vi "oa_Check Data for Waveform Reference (N Channels).vi"(0 "resampled signal":cluster{"r0":dbl, "dr":dbl, "Y":dbl[]}[](array[cluster]) {"r0" format="%.2p"; "dr" format="%.2p"; "Y" format="%.2f"}, 1 "reset? (True)":bool=TRUE, 5 "select reference data":T2(ring), 7 "speed profile":T1 {"speed [RPM]" format="%.2f"; "time [s]" format="%.2f"}, 9 "interpolated pulse positions":dbl[](array[numeric]) format="%.2f", 11 "error in (no error)":errorcluster, 12 "even angle references in":cluster{"r0":dbl, "dr":dbl, "Y":dbl[]}[](array[cluster]) {"r0" format="%.2p"; "dr" format="%.2p"; "Y" format="%.2f"}) -> (2 "empty signal?":bool, 3 "reset":bool, 4 "resampled data out":cluster{"r0":dbl, "dr":dbl, "Y":dbl[]}[](array[cluster]) {"r0" format="%.2p"; "dr" format="%.2p"; "Y" format="%.2f"}, 6 "select reference dataout":T2(ring), 8 "speed profile out":T1 {"speed [RPM]" format="%.2f"; "time [s]" format="%.2f"}, 10 "interpolated pulse positions out":dbl[](array[numeric]) format="%.2f", 14 "even angle references out":cluster{"r0":dbl, "dr":dbl, "Y":dbl[]}[](array[cluster]) {"r0" format="%.2p"; "dr" format="%.2p"; "Y" format="%.2f"}, 15 "error out":errorcluster)   [LabVIEW 2017, in "SoundVib_Resampling.lvlib"]
uses:
  <vilib>/addons/Sound and Vibration/Order Analysis/Resample Order Tracking/SoundVib_Resampling.lvlib
  <vilib>/addons/Sound and Vibration/Order Analysis/Tach Process/SubVIs/speed profile.ctl
  <vilib>/addons/Sound and Vibration/Order Analysis/Resample Order Tracking/SubVIs/OAT Verify Resampled Signal (Multi Channels).vi
  <vilib>/addons/Sound and Vibration/Order Analysis/Tach Process/SoundVib_TachProcess.lvlib
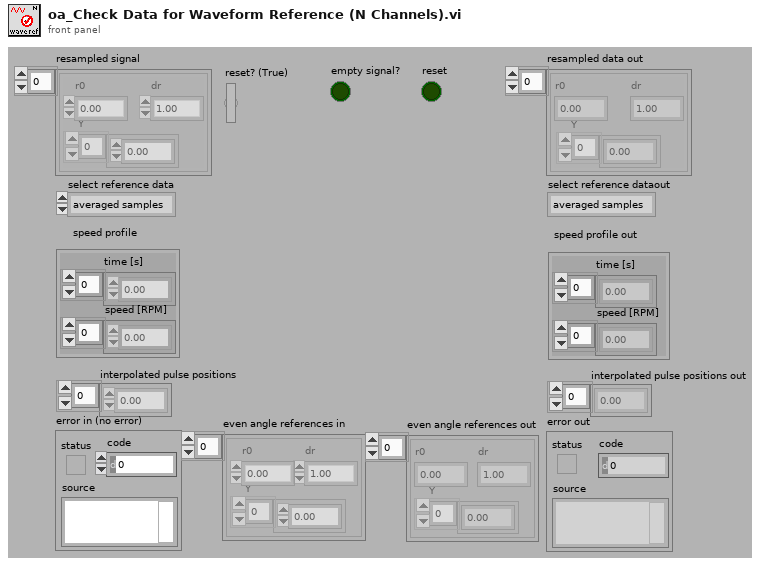
[diagram p1: front panel]
types:
  T1 = typedef "SoundVib_TachProcess.lvlib/speed profile.ctl" = cluster{"time [s]":dbl[], "speed [RPM]":dbl[]}
  T2 = enum16{"averaged samples", "initial samples", "final samples"}
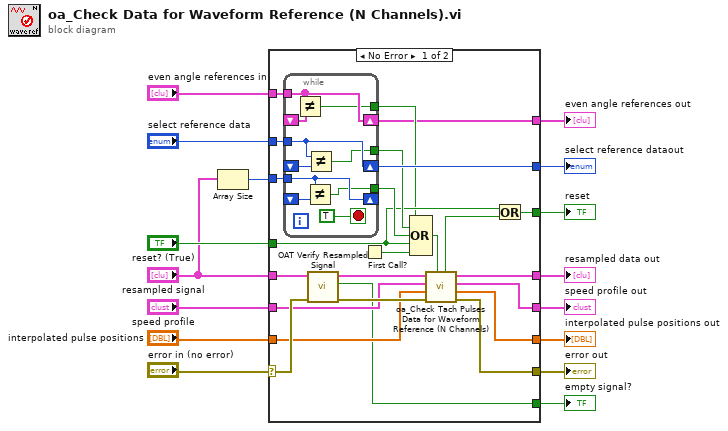
[diagram p0: block diagram]
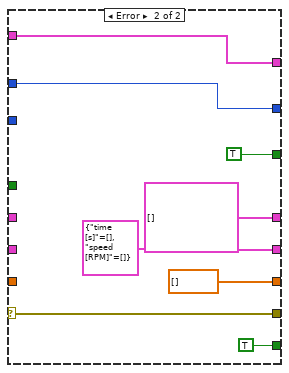
[diagram p2: hidden frame]
diagram:
  n1 = Array Size(array="resampled signal") -> (size(s)=w5:i32)
  n2 = case shown="No Error" "error in (no error)" {
    selector: "error in (no error)" -> [w29 w58]
    tunnel: [w20 w58] -> w11
    tunnel: "select reference data" -> [w40 w57]
    tunnel: "reset? (True)" -> [w35 _]
    tunnel: [w39 w57] -> w7
    tunnel: "resampled signal" -> [w30 _]
    tunnel: "speed profile" -> [w25 _]
    tunnel: "interpolated pulse positions" -> [w24 _]
    tunnel: [w23 cluster{"r0":dbl, "dr":dbl, "Y":dbl[]}[] []] -> w10
    tunnel: [w22 T1 {"time [s]"=[], "speed [RPM]"=[]} ("speed profile out")] -> w9
    tunnel: [w21 dbl[] [] ("interpolated pulse positions out")] -> w8
    tunnel: [w34 TRUE ("reset")] -> w4
    tunnel: w5 -> [w38 _]
    tunnel: "even angle references in" -> [w32 w52]
    tunnel: [w28 w52] -> w2
    tunnel: [w17 TRUE ("empty signal")] -> w1
    frame No Error {
      n3 = while {
        shift-right: [w50] -> w39
        shift-left: _ -> [w47]
        tunnel: w40 -> [w50]
        tunnel: [w48] -> w37
        shift-right: [w45] -> _
        shift-left: _ -> [w46]
        tunnel: w38 -> [w45]
        tunnel: [w44] -> w36
        tunnel: w32 -> [w42]
        shift-right: [w42] -> w28
        shift-left: _ -> [w43]
        tunnel: [w41] -> w31
        stop <- TRUE stop-if-true
        n4 = Not Equal?(x=w42, y=w43) -> (x != y?=w41:bool)
        n5 = Not Equal?(x=w45, y=w46) -> (x != y?=w44:bool)
        n6 = Not Equal?(x=w50, y=w47) -> (x != y?=w48:bool)
      }
      n7 = call-poly <vilib>:"OAT Verify Resampled Signal.vi"("error in (no error)"=w29, "resampled signal"=w30) -> ("error out"=w26:errorcluster, "empty signal"=w17:bool, "resampled signal out"=w27:cluster{"r0":dbl, "dr":dbl, "Y":dbl[]}[])  [unwired: 7 in]
      n8 = First Call?() -> (First Call?: T/F=w33:bool)
      n9 = Compound Arithmetic op=OR(w31, w37, w36, w35, w33) -> (w19:bool)
      n10 = call <vilib>:"oa_Check Tach Pulses Data for Waveform Reference (N Channels).vi"("reset? (True)"=w19, "error in (no error)"=w26, "interpolated pulse positions"=w24, "speed profile"=w25, "even angle signals"=w27) -> ("error out"=w20:errorcluster, "interpolated pulse positions out"=w21:dbl[], "speed profile out"=w22:T1, "even angle signals"=w23:cluster{"r0":dbl, "dr":dbl, "Y":dbl[]}[], "reset"=w18:bool)  [unwired: 2 in]
      n11 = Or(x=w35, y=w18) -> (x .or. y?=w34:bool)
    }
    frame Error {
    }
  }
  "select reference dataout" <- w7
  "interpolated pulse positions out" <- w8
  "speed profile out" <- w9
  "error out" <- w11
  "reset" <- w4
  "resampled data out" <- w10
  "even angle references out" <- w2
  "empty signal?" <- w1
